vi "PadLookupVar.vi"() -> ()   [LabVIEW 2012]
uses:
  Controls/PadLookup.ctl
  Controls/PadLookupItem.ctl
  Controls/PadArea.ctl
panel:
  out "PadLookup":T1
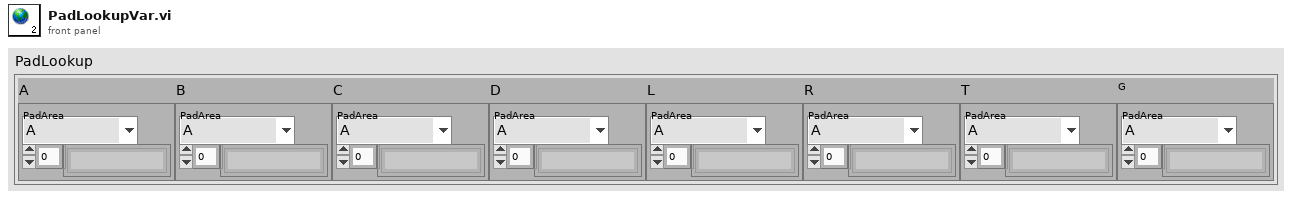
[diagram p1: front panel]
types:
  T1 = typedef "PadLookup.ctl" = cluster{"A":T2, "B":T2, "C":T2, "D":T2, "L":T2, "R":T2, "T":T2, "G":T2}
  T2 = typedef "PadLookupItem.ctl" = cluster{"PadArea":T3, string[]}
  T3 = typedef "PadArea.ctl" = enum16{"A", "B", "C", "D", "L", "R", "T", "G"}
diagram:
